vi "td.vi"() -> ()   [LabVIEW 2018]
panel:
  out "输出":T1(array[cluster])
  in  "簇 4":T2
  in  "簇 3":T3
  in  "簇 2":T3
  in  "簇":T4
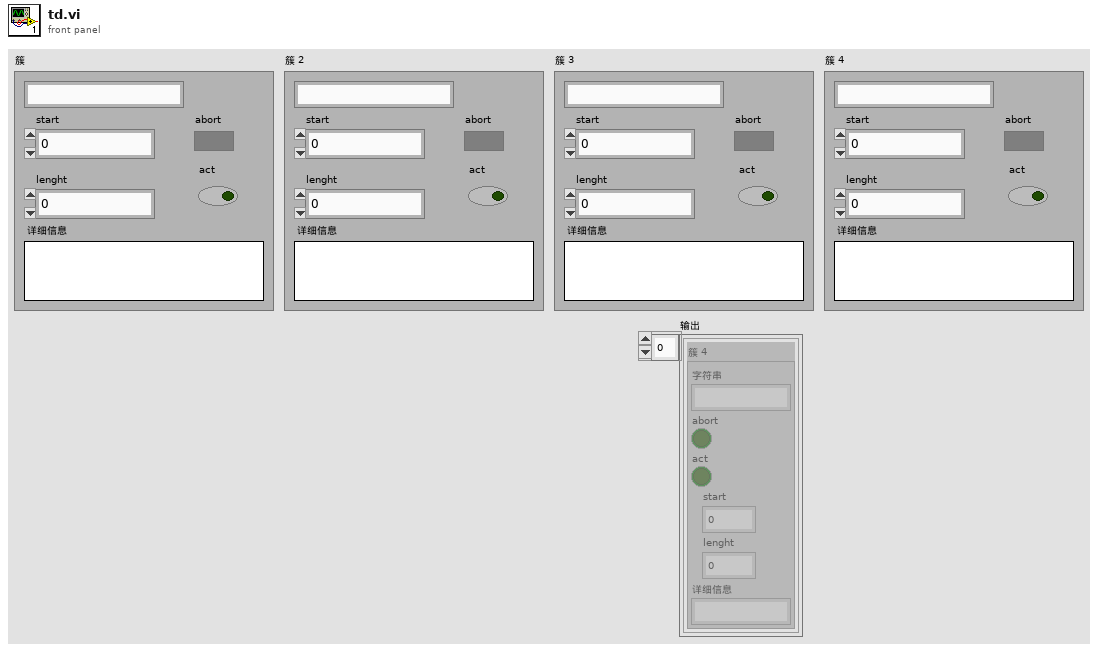
[diagram p1: front panel]
types:
  T1 = cluster{"簇 4":cluster{"字符串":string, "abort":bool, "act":bool, "start":dbl, "lenght":dbl, "详细信息":string}}[]
  T2 = cluster{"字符串":string, "abort":bool, "act":bool, "start":dbl, "lenght":dbl, "详细信息":string}
  T3 = cluster{"title":string, "abort":bool, "act":bool, "start":dbl, "lenght":dbl, "详细信息":string}
  T4 = cluster{"title\ntitle":string, "abort":bool, "act":bool, "start":dbl, "lenght":dbl, "详细信息":string}
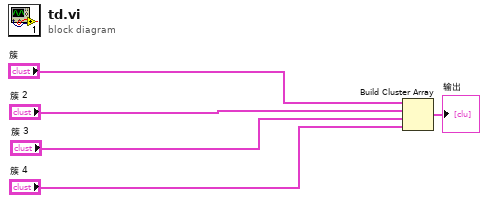
[diagram p0: block diagram]
diagram:
  n1 = Build Cluster Array("簇", "簇 2", "簇 3", "簇 4") -> (→"输出":T1)
